vi "Find record in CSV.vi"(0 "CSV file":path, 5 "Search key":string, 7 "Search key column (0-n)":u32, 9 "Return columns list (commas)":string, 11 "error in":errorcluster) -> (2 "Record match numbers":u32[](array[numeric]), 3 "Record matches":i32, 4 "Record not found?":bool=TRUE, 6 "First column from list":string, 8 "All columns from list":string[](array[string]), 10 "Rows":i32, 13 "Headers":string[](array[string]), 14 "Columns":i32, 15 "error out":errorcluster)   [LabVIEW 2013]
doc: "Pass csv file name with search key and column number with return column list separated by columns (0,2,6). Will return header list from first row/line, column data from first entry in comma separated list so you don't have to index out data if you want just one field, the complete return columns list for all columns you asked for, numbers of matches with record number list, total records (rows) including header row"
uses:
  <vilib>/Utility/file.llb/Read From Spreadsheet File (string).vi
panel:
  out "Spread Sheet Display":string[][](array[string])
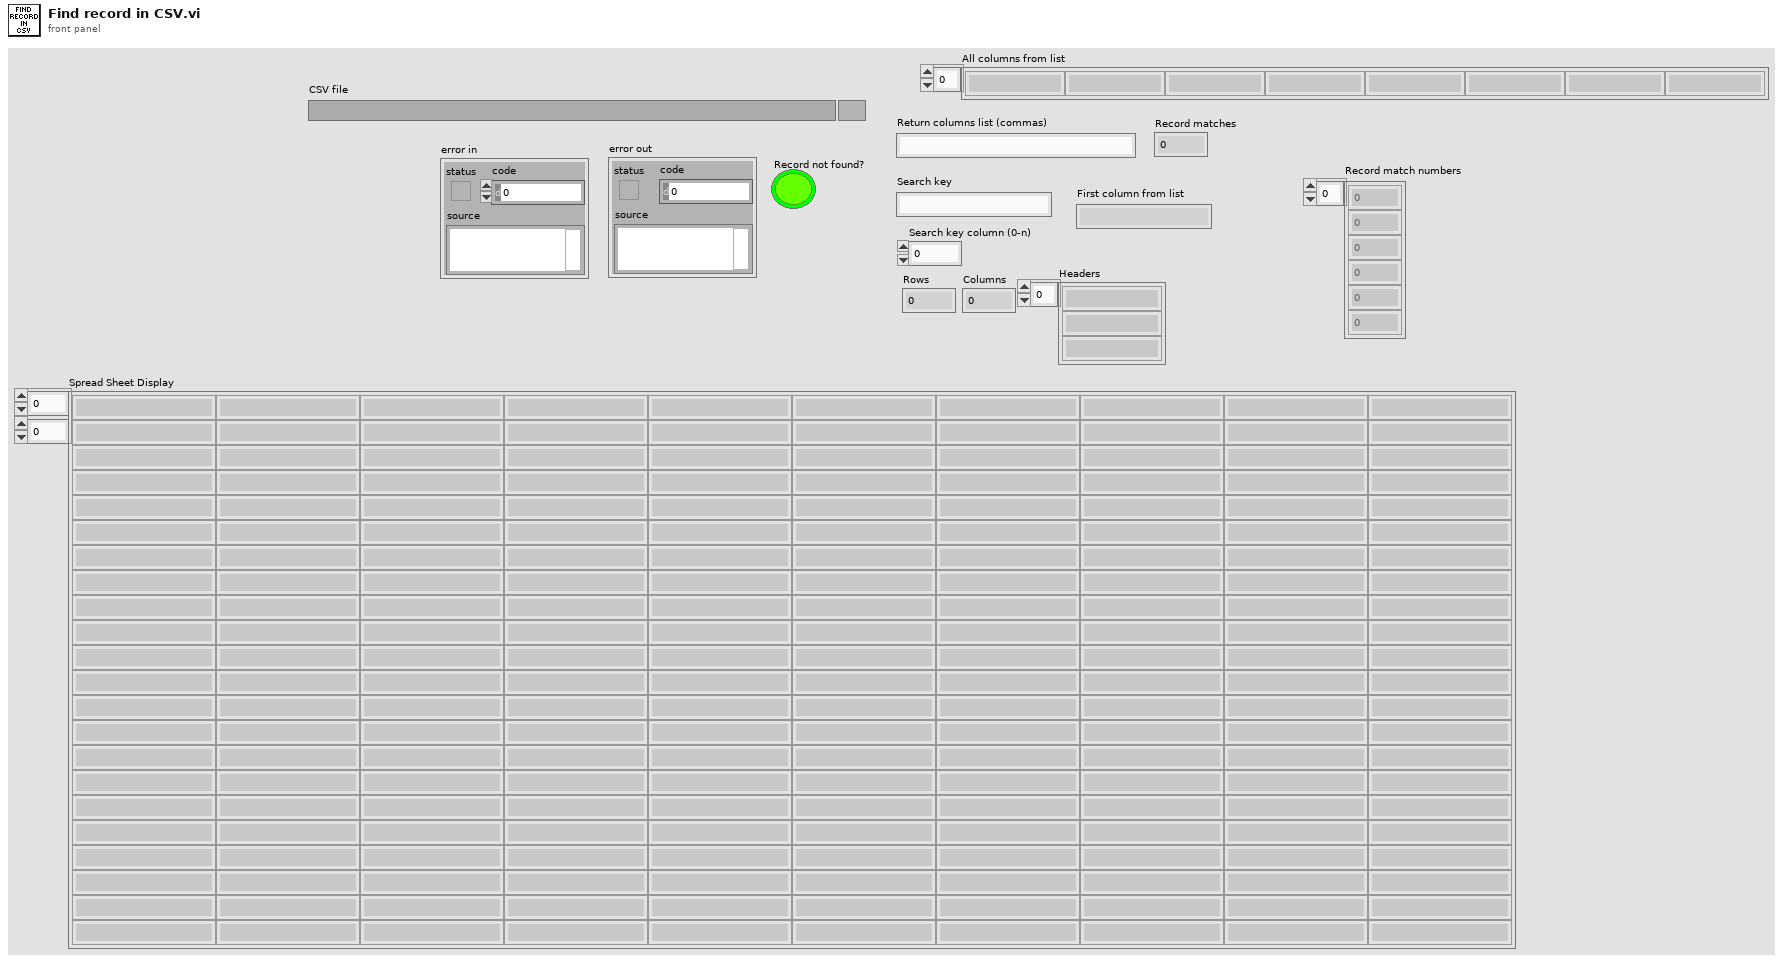
[diagram p1: front panel]
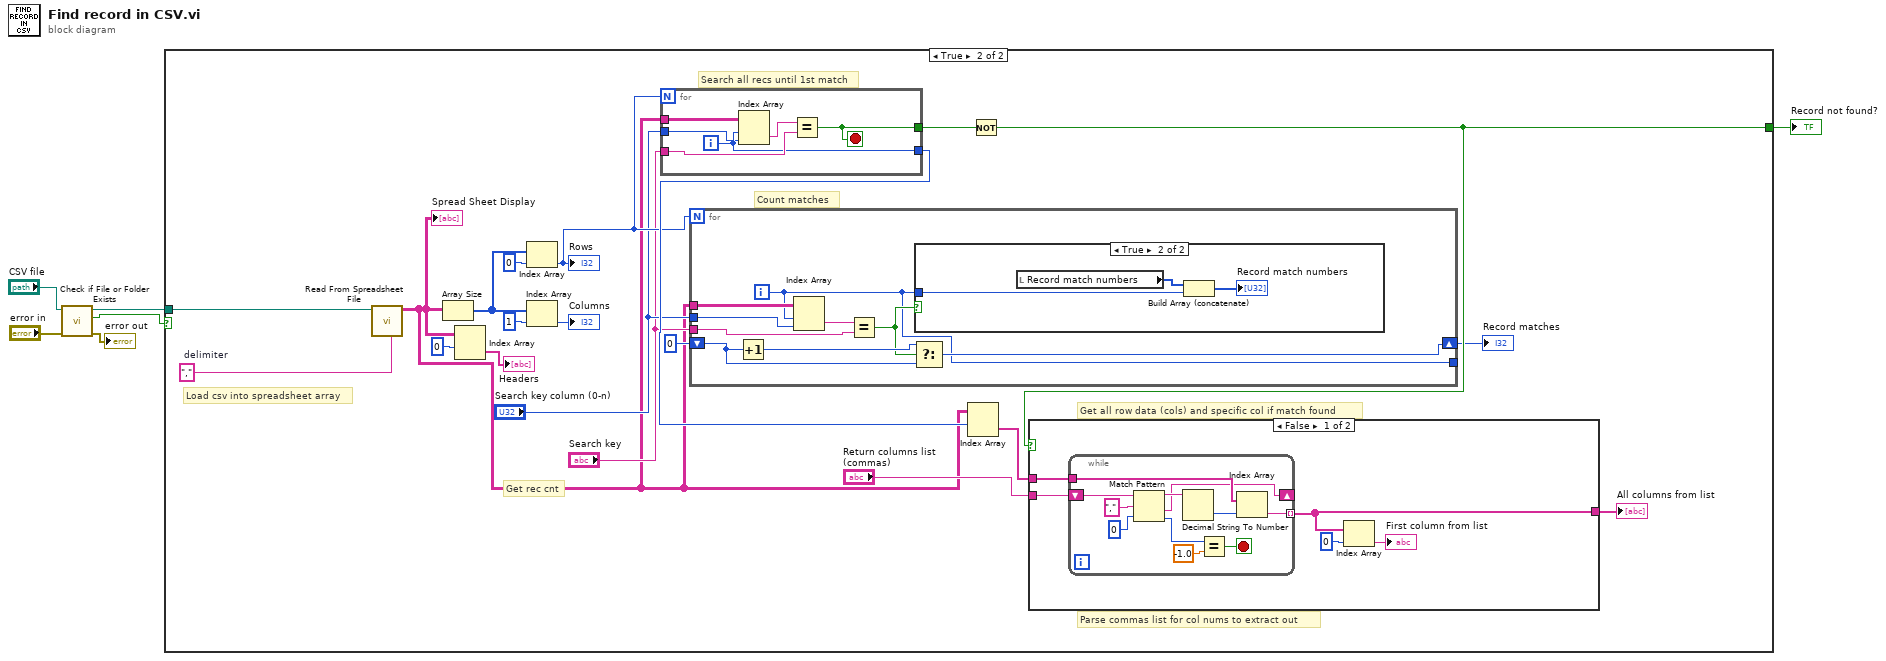
[diagram p0: block diagram]
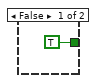
[diagram p2: hidden frame]
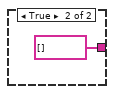
[diagram p4: hidden frame]
diagram:
  n1 = call <vilib>:"Check if File or Folder Exists.vi"("error in (no error)"="error in", "path"="CSV file") -> ("error out"=→"error out":errorcluster, "file or folder exists?"=w4:bool, "dup path"=w1:path)  [unwired: 7 in]
  n2 = case shown="True" w4 {
    tunnel: [TRUE w21] -> w3
    tunnel: w1 -> [_ w24]
    frame False {
    }
    frame True {
      w27 = ","  # delimiter
      # "Count matches"
      # "Parse commas list for col nums to extract out"
      # "Get all row data (cols) and specific col if match found"
      # "Search all recs until 1st match"
      # "Load csv into spreadsheet array"
      # "Get rec cnt"
      n3 = call-poly <vilib>:"Read From Spreadsheet File.vi"("delimiter (\\t)"=w27, "file path (dialog if empty)"=w24) -> ("all rows"=w10:string[][])  [unwired: 5 in, 4 out]
      "Spread Sheet Display" <- w10
      n4 = Array Size(array=w10) -> (size(s)=w17:i32[])
      n5 = Index Array(array=w10, index (row)=0) -> (element=→"Headers":string[])  [unwired: 1 in]
      n6 = Index Array(array=w17, index=0) -> (element=w15:i32)
      "Rows" <- w15
      n7 = Index Array(array=w17, index=1) -> (element=→"Columns":i32)
      n8 = for {
        N: w15 -> [_]
        tunnel: w10 -> [w57]
        tunnel: "Search key" -> [w61]
        tunnel: [w60] -> w20
        tunnel: "Search key column (0-n)" -> [w59]
        tunnel: [w58] -> w25
        i -> [w60]
        stop <- w58 stop-if-true
        n9 = Index Array(array=w57, index (row)=w60, index (col)=w59) -> (element=w62:string)
        n10 = Equal?(x=w62, y=w61) -> (x = y?=w58:bool)
      }
      n11 = for {
        N: w15 -> [_]
        tunnel: w10 -> [w33]
        tunnel: "Search key" -> [w35]
        tunnel: [w28] -> _
        tunnel: "Search key column (0-n)" -> [w34]
        shift-right: [w32] -> w11
        shift-left: 0 -> [w31]
        i -> [w28]
        n12 = Increment(x=w31) -> (x+1=w30:i32)
        n13 = Index Array(array=w33, index (row)=w28, index (col)=w34) -> (element=w36:string)
        n14 = Equal?(x=w36, y=w35) -> (x = y?=w29:bool)
        n15 = Select(t=w30, s=w29, f=w31) -> (s? t:f=w32:i32)
        n16 = case shown="True" w29 {
          tunnel: w28 -> [_ w38]
          frame False {
          }
          frame True {
            n17 = local read "Record match numbers"() -> (w39:u32[])
            n18 = Build Array (concatenate)(w39, w38) -> (→"Record match numbers":u32[])
          }
        }
      }
      "Record matches" <- w11
      n19 = Index Array(array=w10, index (row)=w20) -> (element=w19:string[])  [unwired: 1 in]
      n20 = Not(x=w25) -> (.not. x?=w21:bool)
      n21 = case shown="False" w21 {
        tunnel: "Return columns list (commas)" -> [w44 _]
        tunnel: [w42 string[] [] ("all rows")] -> w22
        tunnel: w19 -> [w43 _]
        frame False {
          n22 = while {
            tunnel: [w50] -> w42 mode=indexing
            tunnel: w43 -> [w49]
            shift-right: [w47] -> _
            shift-left: w44 -> [w55]
            stop <- w53 stop-if-true
            n23 = Match Pattern(string=w55, regular expression=",", offset (0)=0) -> (before substring=w51:string, after substring=w47:string, offset past match=w46:i32)  [unwired: 1 out]
            n24 = Decimal String To Number(string=w51) -> (number=w48:i32)  [unwired: 2 in, 1 out]
            n25 = Equal?(x=w46, y=-1.0) -> (x = y?=w53:bool)
            n26 = Index Array(array=w49, index=w48) -> (element=w50:string)
          }
          n27 = Index Array(array=w42, index=0) -> (element=→"First column from list":string)
        }
        frame True {
        }
      }
      "All columns from list" <- w22
    }
  }
  "Record not found?" <- w3
